vi "Initialize Write Data to VS Engine.vi"(7 "Name":string, 8 "error in (no error)":errorcluster, 9 "FIFO Name":string, 10 "Hardware Output Refs":T1[](array[typedef]) format="%.0x", 11 "Device Ref":T1 format="%.0x") -> (0 "error out":errorcluster, 2 "Write to VS Engine":T2 {"Pairs"."Refs" format="%.0x"}, 3 "Device Ref out":T1=18446744073709551615 format="%.0x")   [LabVIEW 2015, in "Control Addon Engine.lvlib" / "Inline Async API.lvlib"]
uses:
  Inline Async API.lvlib
  Controls/Write To VS Engine.ctl
  <vilib>/NI Veristand/Custom Device API/Data Reference.ctl
  <vilib>/NI Veristand/Custom Device API/Custom Device Item Ref.ctl
  <vilib>/NI Veristand/Custom Device API/Data Access Type.ctl
  <vilib>/NI VeriStand/Custom Device API/Custom Device API.lvlib
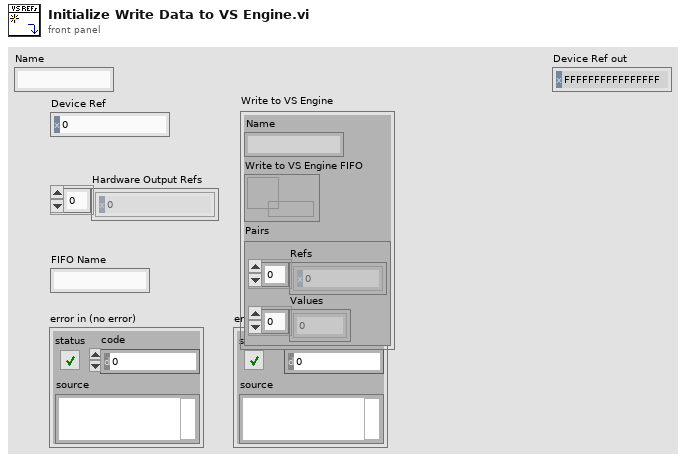
[diagram p1: front panel]
types:
  T1 = typedef "Custom Device API.lvlib/Custom Device Item Ref.ctl" = u64
  T2 = typedef "Control Addon Engine.lvlib/Inline Async API.lvlib/Write To VS Engine.ctl" = cluster{"Name":string, "Write to VS Engine FIFO":refnum<k33>, "Pairs":cluster{"Refs":T3[], "Values":dbl[]}}
  T3 = typedef "Custom Device API.lvlib/Data Reference.ctl" = i32
  T4 = typedef "Custom Device API.lvlib/Data Access Type.ctl" = enum16{"Read", "Write"}
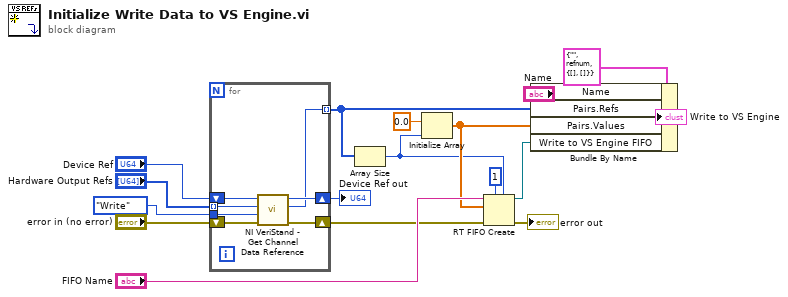
[diagram p0: block diagram]
diagram:
  n1 = for {
    tunnel: "Hardware Output Refs" -> [w20] mode=indexing
    tunnel: Data_Access_Type."Write" ("Access") -> [w19]
    shift-right: [w22] -> w6
    shift-left: "error in (no error)" -> [w23]
    shift-right: [w24] -> w3
    shift-left: "Device Ref" -> [w21]
    tunnel: [w18] -> w4 mode=indexing
    n2 = call <vilib>:"NI VeriStand - Get Channel Data Reference.vi"("error in (no error)"=w23, "Access"=w19, "Channel Ref in"=w20, "Device Ref in"=w21) -> ("error out"=w22:errorcluster, "Channel Data Reference"=w18:T3, "Device Ref out"=w24:T1)  [unwired: 5 in]
  }
  "Device Ref out" <- w3
  n3 = Array Size(array=w4) -> (size(s)=w10:i32)
  n4 = Initialize Array(0.0 ("element"), w10) -> (w13:dbl[])
  n5 = RT FIFO Create(0:"FIFO Name", 1:w13, 3:w6, 4:u32 1 ("size (10)"), 6:w10) -> (8:w14:refnum<k33>, 11:→"error out":errorcluster)  [unwired: 3 in, 1 out]
  n6 = Bundle By Name(cluster=T2 {"Name"="", "Write to VS Engine FIFO"=refnum, "Pairs"={"Refs"=[], "Values"=[]}} ("Write to VS Engine"), "Name"="Name", "Pairs.Refs"=w4, "Pairs.Values"=w13, "Write to VS Engine FIFO"=w14) -> (→"Write to VS Engine":T2)
